vi "Robot Systems.vi"(11 "output cluster":T1) -> ()   [LabVIEW 2016]
uses:
  Joystick/ControlsToCommands.ctl
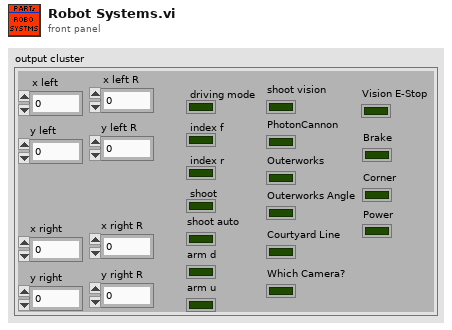
[diagram p1: front panel]
types:
  T1 = typedef "ControlsToCommands.ctl" = cluster{"x left":dbl, "y left":dbl, "x right":dbl, "y right":dbl, "driving mode":bool, "index f":bool, "index r":bool, "shoot":bool, "shoot auto":bool, "arm d":bool, "arm u":bool, "shoot vision":bool, "PhotonCannon":bool, "Outerworks":bool, "Outerworks Angle":bool, "Courtyard Line":bool, "Which Camera?":bool, "Vision E-Stop":bool, "x left R":dbl, "y left R":dbl, "x right R":dbl, "y right R":dbl, "Brake":bool, "Corner":bool, "Power":bool}
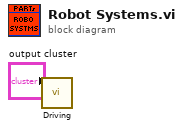
[diagram p0: block diagram]
diagram:
  n1 = call "Driving.vi"("output cluster"="output cluster") -> ()  [unwired: 11 in]
